vi "SplitString(SubVI).vi"(11 "data in":string) -> (0 "Numeric":dbl, 3 "String 3":string)   [LabVIEW 2016]
panel:
  out "value":dbl
  out "match + rest of string":string
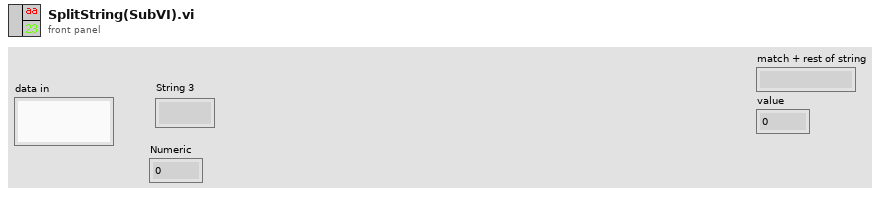
[diagram p1: front panel]
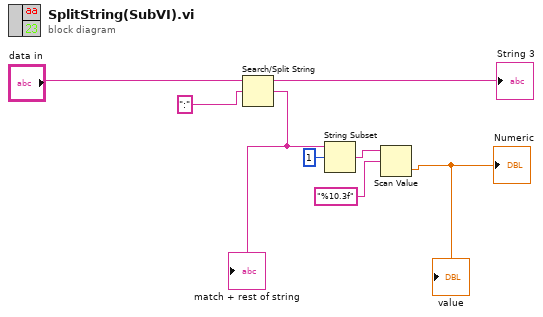
[diagram p0: block diagram]
diagram:
  n1 = Search/Split String(string="data in", search string/char (-)=":") -> (substring before match=→"String 3":string, match + rest of string=w3:string)  [unwired: 1 in, 1 out]
  "match + rest of string" <- w3
  n2 = String Subset(string=w3, offset (0)=1) -> (substring=w1:string)  [unwired: 1 in]
  n3 = Scan Value(string=w1, format string="%10.3f") -> (value=→"Numeric" →"value":dbl)  [unwired: 1 in, 1 out]
